vi "Poll Raw Wrapper.vi"(8 "error in (no error)":errorcluster, 10 "Buffer in":u8[](array[numeric])=[0, 0, 0, 0, 0, 0, 0, 0, 0, 0, 0, 0, 0, 0, 0, 0, 0, 0, 0, 0, 0, 0, 0, 0, 0, 0, 0, 0, 0, 0, 0, 0] format="%.0x", 11 "Reader Handle":i64) -> (0 "error out":errorcluster, 1 "Timeout":bool, 2 "Buffer Out":u8[](array[numeric]) format="%.0x", 3 "Valid Bytes":u64)   [LabVIEW 2021, in "Zenoh.lvclass"]
uses:
  Zenoh.lvclass
  Zenoh.lvclass/Zenoh.ctl
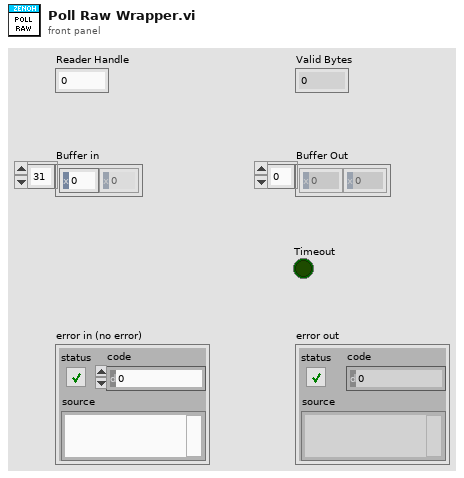
[diagram p1: front panel]
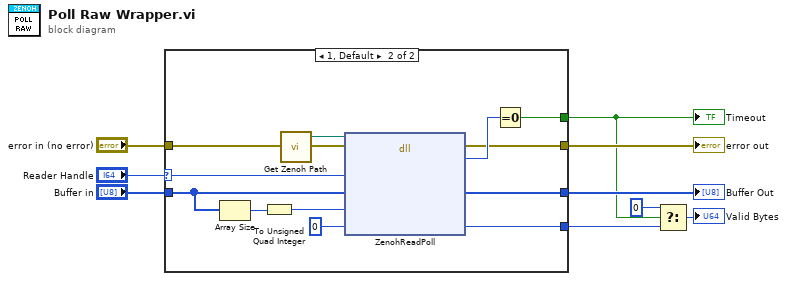
[diagram p0: block diagram]
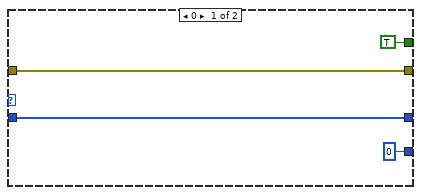
[diagram p2: hidden frame]
diagram:
  n1 = case shown="1, Default" "Reader Handle" {
    selector: "Reader Handle" -> [_ w22]
    tunnel: [w13 w16] -> w9
    tunnel: "error in (no error)" -> [w13 w23]
    tunnel: "Buffer in" -> [w12 w19]
    tunnel: [TRUE w17] -> w3
    tunnel: [u64 0 ("actualLen") w15] -> w4
    tunnel: [w12 w14] -> w5
    frame 0 {
    }
    frame 1, Default {
      n2 = Array Size(array=w19) -> (size(s)=w25:i32)
      n3 = To Unsigned Quad Integer(1:w25) -> (0:w20:u64)
      n4 = call "Get Zenoh Path.vi"() -> ("Library Path"=w21:path)  [unwired: 4 in]
      n5 = dll-call lib="D:/dev/zenoh/wrapper/zenoh_wrapper_reader.dll" fn="ZenohReadPoll"(path in=w21, error in=w23, "readerHandle"=w22, "buffer"=w19, "bufferMax"=w20, "actualLen"=u64 0) -> (error out=w16:errorcluster, "return type"=w18:i32, "buffer"=w14:u8[], "actualLen"=w15:u64)  [unwired: 3 in, 1 out]
      n6 = Equal To 0?(x=w18) -> (x = 0?=w17:bool)
    }
  }
  "error out" <- w9
  "Timeout" <- w3
  "Buffer Out" <- w5
  n7 = Select(t=u64 0, s=w3, f=w4) -> (s? t:f=→"Valid Bytes":u64)
